vi "Update Node Info.vi"(8 "error in (no error)":errorcluster, 10 "Node Info":T1, 11 "InfoService in":refnum<class "InfoService.lvclass">) -> (0 "error out":errorcluster, 3 "InfoService out":refnum<class "InfoService.lvclass">)   [LabVIEW 2020, in "Vecto.lvlib" / "InfoService.lvclass"]
uses:
  InfoService.lvclass
  Node Info.ctl
  Task Info.ctl
  Node Info Data'.ctl
  InfoService.lvclass/InfoService.ctl
  Vecto.lvlib
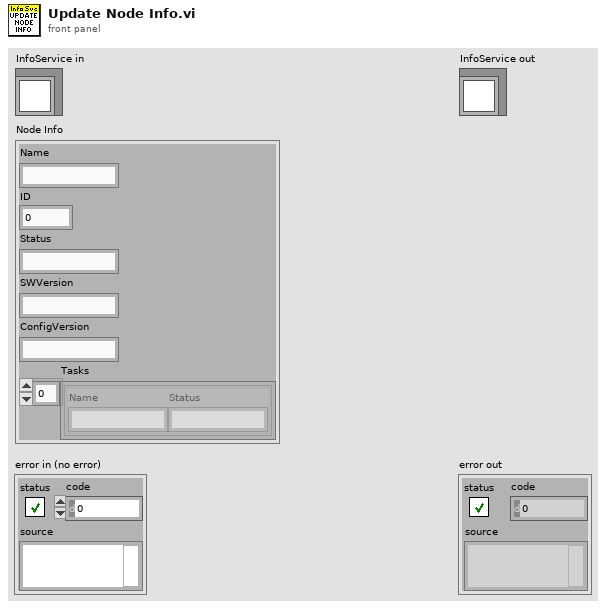
[diagram p1: front panel]
types:
  T1 = typedef "Vecto.lvlib/Node Info.ctl" = cluster{"Name":string, "ID":i32, "Status":string, "SWVersion":string, "ConfigVersion":string, "Tasks":T2[]}
  T2 = typedef "Vecto.lvlib/Task Info.ctl" = cluster{"Name":string, "Status":string}
  T3 = typedef "Vecto.lvlib/InfoService.lvclass/Node Info Data'.ctl" = cluster{"Node Info":T1}
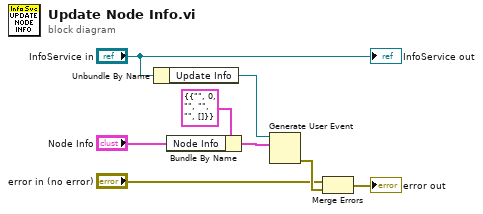
[diagram p0: block diagram]
diagram:
  n1 = Unbundle By Name("InfoService in") -> ("Update Info"=w8:refnum<user-event>)
  n2 = Bundle By Name(cluster=T3 {"Node Info"={"Name"="", "ID"=0, "Status"="", "SWVersion"="", "ConfigVersion"="", "Tasks"=[]}} ("event data"), "Node Info"="Node Info") -> (w6:T3)
  n3 = Generate User Event(user event=w8, event data cluster=w6) -> (error out=w4:errorcluster)  [unwired: 2 in, 1 out]
  n4 = Merge Errors("error in (no error)", w4) -> (→"error out":errorcluster)
  "InfoService out" <- "InfoService in"
